vi "系统日志.vi"(11 "data in":T1={"时间"=timestamp(0 s since 1904-01-01), "参数"="系统", "日志信息"="", "流程参数"=""}) -> ()   [LabVIEW 2016]
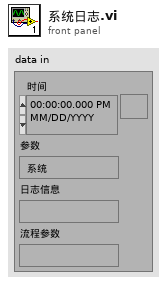
[diagram p1: front panel]
types:
  T1 = typedef "操作日志字段定义.ctl" = cluster{"时间":timestamp, "参数":string, "日志信息":string, "流程参数":string}
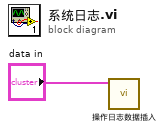
[diagram p0: block diagram]
diagram:
  n1 = call "操作日志数据插入.vi"("data"="data in") -> ()  [unwired: 9 in, 1 out]
